vi "Real_Time_State_Machine.vi"() -> ()   [LabVIEW 2019]
uses:
  <vilib>/Platform/TimedLoop/XDataNode/wakeup.ctl
  <vilib>/Platform/TimedLoop/XDataNode/XDNodeRunTimeDep.lvlib
  <vilib>/Platform/TimedLoop/XDataNode/nitl_modes.ctl
  <vilib>/Platform/TimedLoop/XDataNode/timing_clust.ctl
  <vilib>/platform/TimedLoop/XDataNode/XDataNode.xnode
  <vilib>/myRIO/Common/Instrument Driver Framework/myRIO v1.0/Accelerometer/typedefs/Accelerometer Channels Enum.ctl
  <vilib>/myRIO/Common/Instrument Driver Framework/myRIO v1.0/Accelerometer/typedefs/Accelerometer Channels List.ctl
  <vilib>/myRIO/Common/Instrument Driver Framework/Utilities/typedefs/Generic FPGA Reference.ctl
  <vilib>/myRIO/Common/Instrument Driver Framework/Utilities/typedefs/myRIO v1.0 Reference.ctl
  <vilib>/myRIO/Common/Instrument Driver Framework/Utilities/typedefs/Hardware Version Enum.ctl
  <vilib>/myRIO/Common/Instrument Driver Framework/Utilities/typedefs/myRIO Generic Hardware Reference.ctl
  <vilib>/myRIO/Instrument Drivers/Onboard Devices/Accelerometer/typedefs/Accelerometer Reference.ctl
  <vilib>/myRIO/Instrument Drivers/Onboard Devices/Accelerometer/Accelerometer.lvlib
  <vilib>/myRIO/Instrument Drivers/Onboard Devices/Accelerometer/vis/Read.vi
  <vilib>/userDefined/High Color/nirio_resource_hc.ctl
  <vilib>/myRIO/Instrument Drivers/Onboard Devices/Accelerometer/vis/myRIO Accelerometer Open.xnode
  <vilib>/myRIO/Common/Instrument Driver Framework/Utilities/vis/Is FPGA Ref Available.vi
  <vilib>/myRIO/Express VI/Onboard Devices/Accelerometer/Accelerometer Express VI.xnode
  <vilib>/myRIO/Common/Instrument Driver Framework/myRIO v1.0/DIO/typedefs/DIO Channels Enum.ctl
  <vilib>/myRIO/Common/Instrument Driver Framework/myRIO v1.0/DIO/typedefs/DIO Channels List.ctl
  <vilib>/myRIO/Instrument Drivers/Onboard IO/DIO/typedefs/DIO Reference.ctl
  <vilib>/myRIO/Instrument Drivers/Onboard IO/DIO/DIO.lvlib
  <vilib>/myRIO/Instrument Drivers/Onboard IO/DIO/vis/myRIO DIO Open.xnode
  <vilib>/myRIO/Instrument Drivers/Onboard IO/DIO/vis/Write.vi
  <vilib>/myRIO/Express VI/Onboard Devices/LED/LED Express VI.xnode
  <vilib>/myRIO/Common/Instrument Driver Framework/myRIO v1.0/Accelerometer/vis/myRIO v1.1 Open Accelerometer.vi
  <vilib>/myRIO/Common/Instrument Driver Framework/myRIO v1.0/DIO/vis/myRIO v1.1 Open DIO.vi
  System_State.ctl
  Triggered_State.ctl
  Armed_States.ctl
  Reset_State.ctl
panel:
  in  "Boolean":bool
  in  "Enum 4":T1
  in  "Enum 2":T2
  in  "Enum 3":T3
  in  "Enum":T4=enum."Idle"
  out "Magnitude":dbl
  in  "stop 2":bool
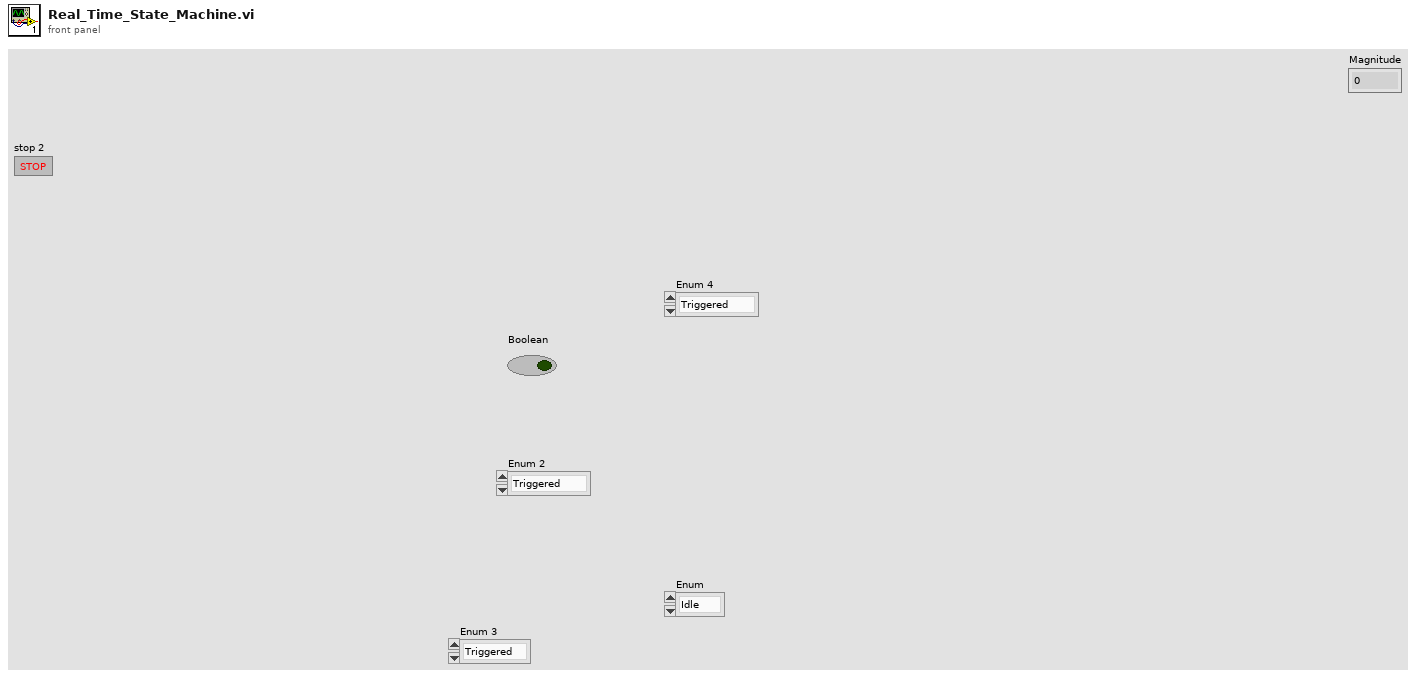
[diagram p1: front panel]
types:
  T1 = typedef "Reset_State.ctl" = enum16{"Triggered", "Armed", "Idle"}
  T2 = typedef "Armed_States.ctl" = enum16{"Triggered", "Armed", "Idle"}
  T3 = typedef "Triggered_State.ctl" = enum16{"Triggered", "Armed", "Idle"}
  T4 = typedef "System_State.ctl" = enum16{"Triggered", "Armed", "Idle"}
  T5 = typedef "XDNodeRunTimeDep.lvlib/timing_clust.ctl" = cluster{"Expected End [f-1]":u64, "Actual End [f-1]":u64, "Finished Late? [f-1]":bool, "Expected End [i-1]":u64, "Actual End [i-1]":u64, "Finished Late? [i-1]":bool, "Expected Start [i]":u64, "Actual Start [i]":u64, "Expected Start [f]":u64, "Actual Start [f]":u64, "Source Name":string, "Structure Name":string, "Period":i64, "Deadline":i64, "Offset":i64, "Start":i64, "Priority":i32, "Timeout":i32, "Mode":T6, "Wakeup Reason":T7, "Error":errorcluster, "Source Type":string, "Secondary Source Type":string, "Global End Time":u64, "Global Start Time":u64, "Frame Duration":u64, "Iteration Duration":u64, "Assigned CPU":i32, "I/O Scan Engine Mode":u32}
  T6 = typedef "XDNodeRunTimeDep.lvlib/nitl_modes.ctl" = enum32{"No Change", "Process missed periods, maintain original phase", "Discard missed periods, maintain original phase", "Process missed periods, ignore original phase", "Discard missed periods, ignore original phase"}
  T7 = typedef "XDNodeRunTimeDep.lvlib/wakeup.ctl" = enum32{"Normal", "Aborted", "Asynchronous wakeup", "Timing source error", "Timed loop error", "Timeout"}
  T8 = typedef "DIO.lvlib/DIO Reference.ctl" = cluster{"myRIO Reference":T9, "DIO Channels List":T13}
  T9 = typedef "myRIO Generic Hardware Reference.ctl" = cluster{"myRIO Model":T10, "myRIO Hardware Reference":T11}
  T10 = typedef "Hardware Version Enum.ctl" = enum16{"Unknown", "myRIO-1900", "myRIO-1950", "roboRIO", "NI ELVIS RIO CM", "ELVIS III"}
  T11 = typedef "myRIO v1.0 Reference.ctl" = cluster{"Generic FPGA Reference":T12, "Allow multiple opens":bool}
  T12 = typedef "Generic FPGA Reference.ctl" = refnum<k20>
  T13 = typedef "DIO Channels List.ctl" = T14[]
  T14 = typedef "DIO Channels Enum.ctl" = enum16{"Not Connected", "C/DIO0", "C/DIO1", "C/DIO2", "C/DIO3", "C/DIO4", "C/DIO5", "C/DIO6", "C/DIO7", "A/DIO0", "A/DIO1", "A/DIO2", "A/DIO3", "A/DIO4", "A/DIO5", "A/DIO6", "A/DIO7", "A/DIO8", "A/DIO9", "A/DIO10", "A/DIO11", "A/DIO12", "A/DIO13", "A/DIO14", "A/DIO15", "A/DIO16", "A/DIO17", "A/DIO18", "A/DIO19", "B/DIO0", "B/DIO1", "B/DIO2", "B/DIO3", "B/DIO4", "B/DIO5", "B/DIO6", "B/DIO7", "B/DIO8", "B/DIO9", "B/DIO10", "B/DIO11", "B/DIO12", "B/DIO13", "B/DIO14", "B/DIO15", "B/DIO16", "B/DIO17", "B/DIO18", "B/DIO19", "LED0", "LED1", "LED2", "LED3", "Button0", "DIO/DIO0", "DIO/DIO1", "DIO/DIO2", "DIO/DIO3", "DIO/DIO4", "DIO/DIO5", "DIO/DIO6", "DIO/DIO7", "DIO/DIO8", "DIO/DIO9", "SPI/CS0", "SPI/CS1", "SPI/CS2", "SPI/CS3", "LED RADIO (Green)", "LED RADIO (Red)", "LED COMM (Green)", "LED COMM (Red)", "LED MODE (Green)", "LED MODE (Red)"}
  T15 = typedef "nirio_resource_hc.ctl" = tag
  T16 = typedef "Accelerometer.lvlib/Accelerometer Reference.ctl" = cluster{"myRIO Reference":T9, "Accelerometer Channels List":T17, "LSB Weight":dbl}
  T17 = typedef "Accelerometer Channels List.ctl" = T18[]
  T18 = typedef "Accelerometer Channels Enum.ctl" = enum16{"Not Connected", "X-Axis", "Y-Axis", "Z-Axis"}
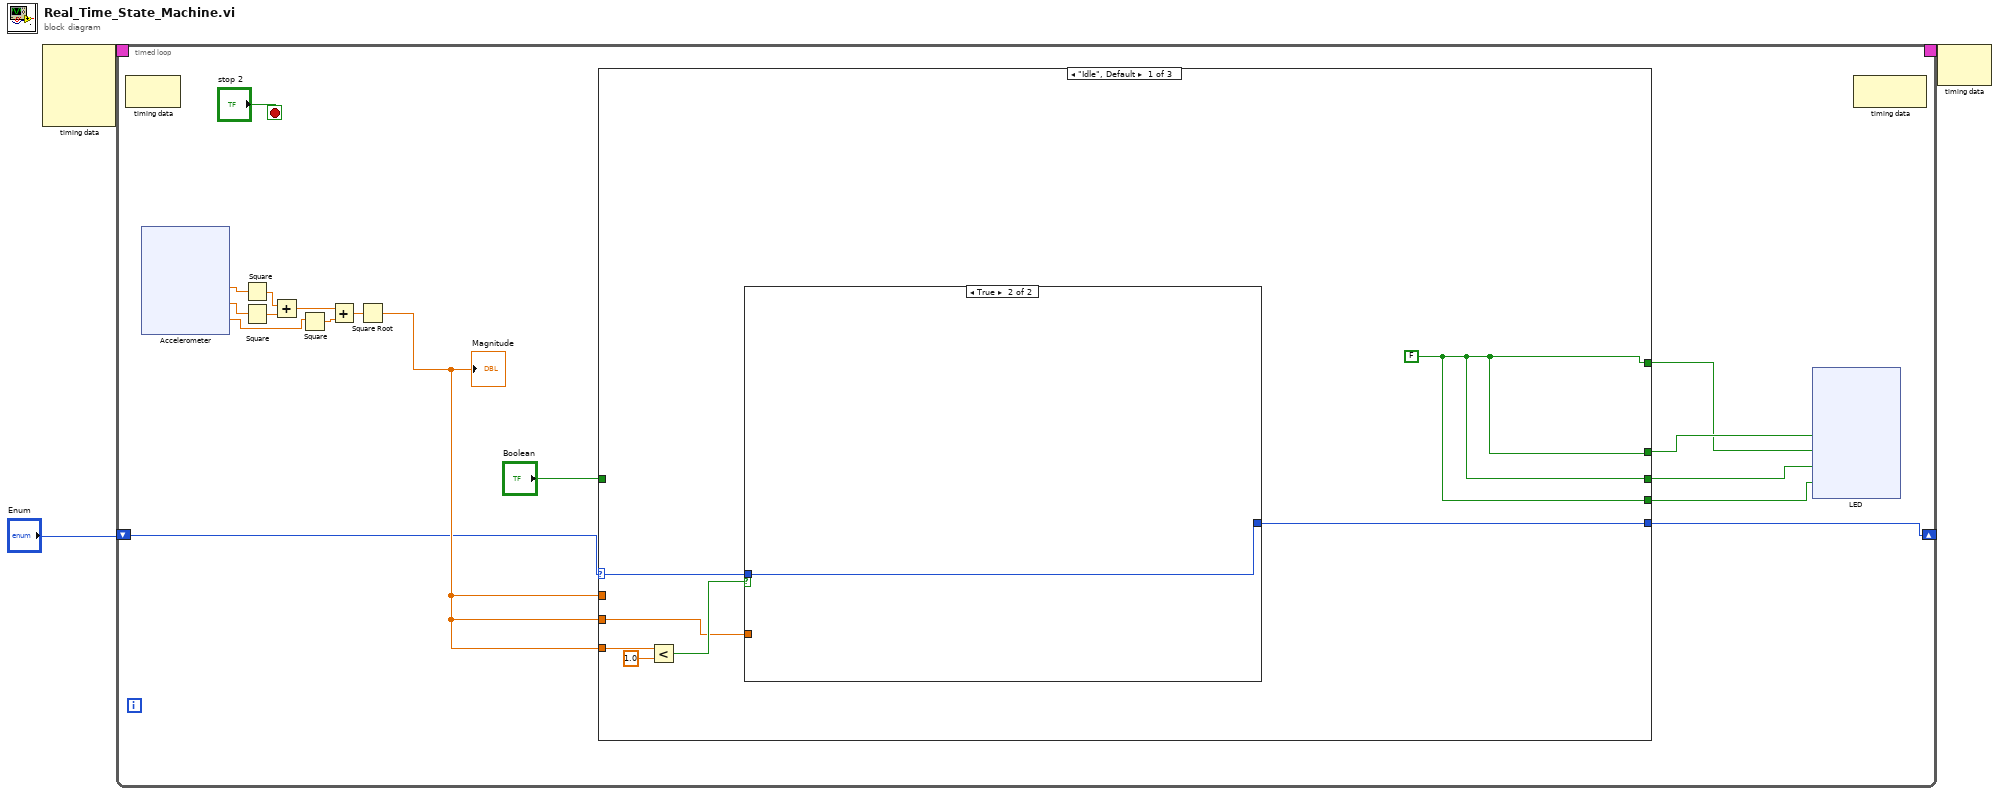
[diagram p0: block diagram]
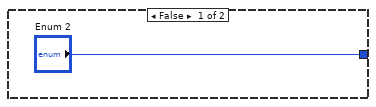
[diagram p2: hidden frame]
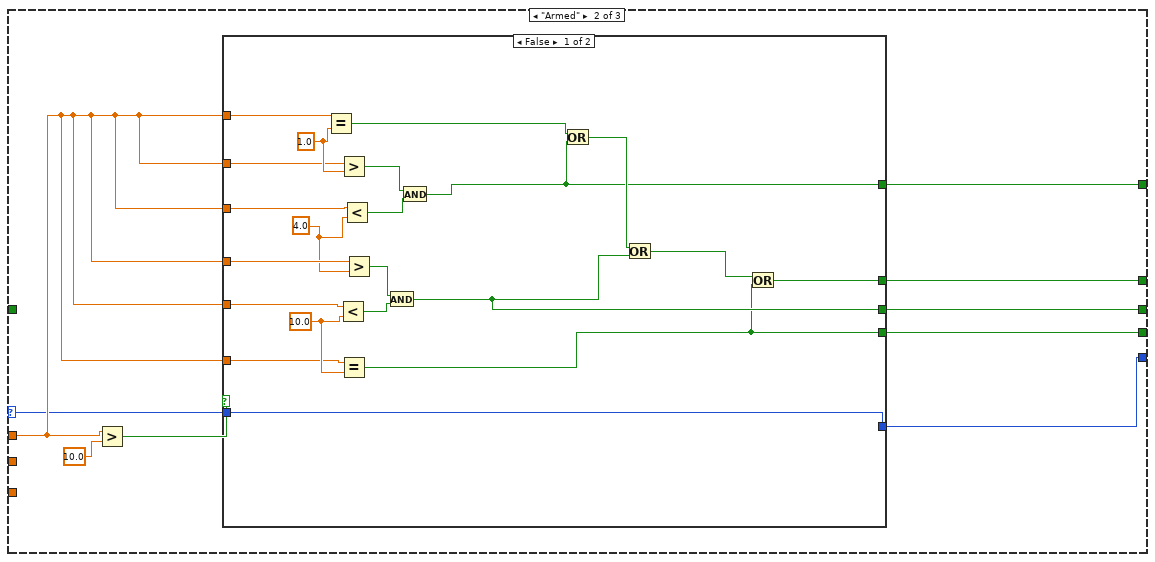
[diagram p3: hidden frame]
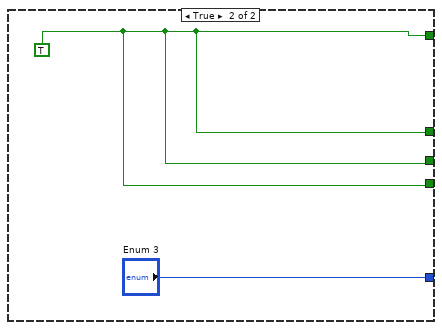
[diagram p4: hidden frame]
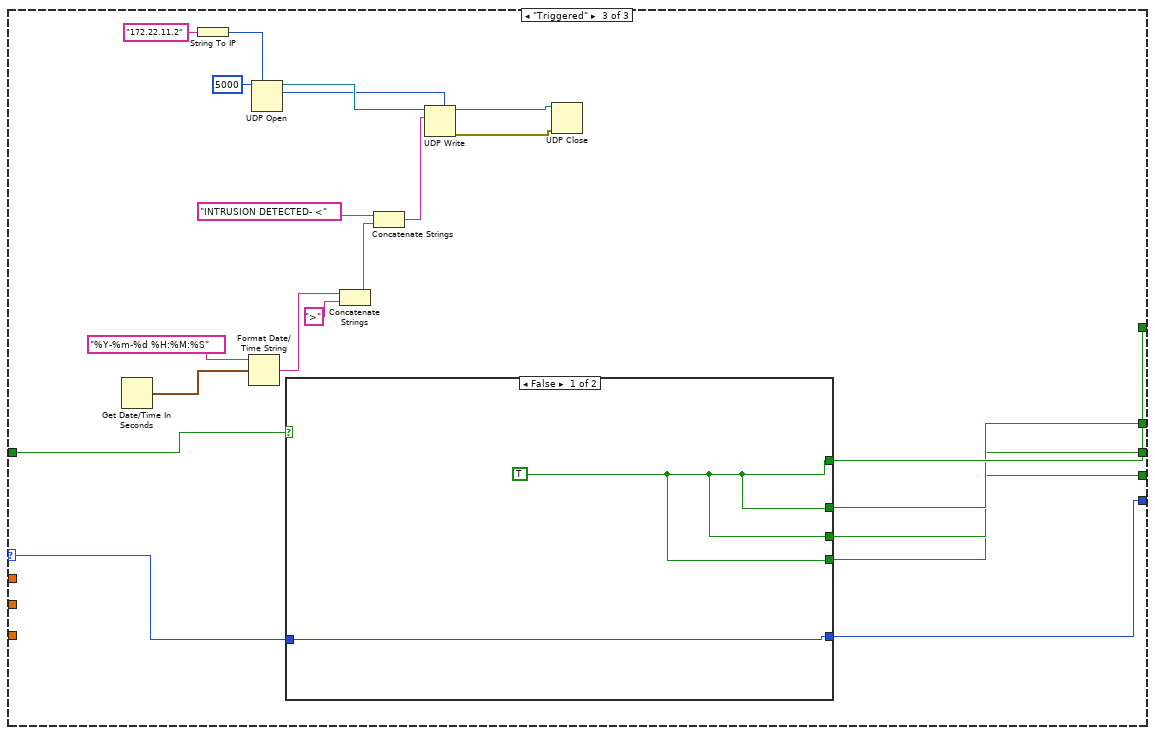
[diagram p5: hidden frame]
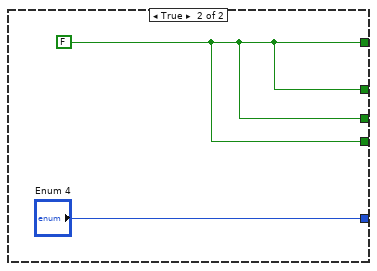
[diagram p6: hidden frame]
diagram:
  n1 = node-c288() -> (w3:T5)  [unwired: 4 in]
  n2 = timed-loop {
    timing: w3 -> [_]
    timing-out: [_] -> w2
    shift-right: [w5] -> _
    shift-left: "Enum" -> [w6]
    stop <- "stop 2" stop-if-true
    n3 = node-c288() -> ()  [unwired: 1 in, 1 out]
    n4 = xnode "Accelerometer"() -> ("X-Axis"=w19:dbl, "Y-Axis"=w18:dbl, "Z-Axis"=w17:dbl)  [unwired: 1 in, 1 out]
    n5 = Square(x=w19) -> (x^2=w16:dbl)
    n6 = Square(x=w18) -> (x^2=w15:dbl)
    n7 = Add(x=w16, y=w15) -> (x+y=w14:dbl)
    n8 = Square(x=w17) -> (x^2=w13:dbl)
    n9 = Add(x=w14, y=w13) -> (x+y=w12:dbl)
    n10 = Square Root(x=w12) -> (sqrt(x)=w11:dbl)
    "Magnitude" <- w11
    n11 = case shown="\"Idle\", Default" w6 {
      selector: w6 -> [w59 w68 w114]
      tunnel: w11 -> [w64 _ _]
      tunnel: w11 -> [w62 _ _]
      tunnel: w11 -> [_ w74 _]
      tunnel: [w61 w73 w118] -> w10
      tunnel: [w61 w72 w119] -> w9
      tunnel: [w61 w71 w117] -> w8
      tunnel: [w61 w70 w116] -> w7
      tunnel: [w60 w69 w115] -> w5
      tunnel: "Boolean" -> [_ _ w120]
      frame "Idle", Default {
        w61 = FALSE
        n12 = Less?(x=w64, y=1.0) -> (x < y?=w63:bool)
        n13 = case shown="True" w63 {
          tunnel: w62 -> [_ _]
          tunnel: ["Enum 2" w67] -> w60
          tunnel: w59 -> [_ w67]
          frame False {
          }
          frame True {
          }
        }
      }
      frame "Armed" {
        n14 = Greater?(x=w74, y=10.0) -> (0:w75:bool)
        n15 = case shown="False" w75 {
          tunnel: w74 -> [w97 _]
          tunnel: w74 -> [w95 _]
          tunnel: w74 -> [w91 _]
          tunnel: w74 -> [w94 _]
          tunnel: w74 -> [w88 _]
          tunnel: w74 -> [w85 _]
          tunnel: [w81 w99] -> w73
          tunnel: [w80 w99] -> w72
          tunnel: [w79 w99] -> w71
          tunnel: [w78 w99] -> w70
          tunnel: [w77 "Enum 3"] -> w69
          tunnel: w68 -> [w77 _]
          frame False {
            w86 = 10.0 ("y")
            w90 = 4.0 ("y")
            w96 = 1.0 ("y")
            n16 = Equal?(x=w97, y=w96) -> (x = y?=w84:bool)
            n17 = Less?(x=w88, y=w86) -> (x < y?=w87:bool)
            n18 = Greater?(x=w95, y=w96) -> (0:w93:bool)
            n19 = Equal?(x=w85, y=w86) -> (x = y?=w78:bool)
            n20 = Less?(x=w91, y=w90) -> (x < y?=w89:bool)
            n21 = Greater?(x=w94, y=w90) -> (0:w92:bool)
            n22 = And(x=w92, y=w87) -> (x .and. y?=w79:bool)
            n23 = And(x=w93, y=w89) -> (x .and. y?=w80:bool)
            n24 = Or(x=w84, y=w80) -> (x .or. y?=w83:bool)
            n25 = Or(x=w83, y=w79) -> (x .or. y?=w82:bool)
            n26 = Or(x=w82, y=w78) -> (x .or. y?=w81:bool)
          }
          frame True {
            w99 = TRUE
          }
        }
      }
      frame "Triggered" {
        n27 = Get Date/Time In Seconds() -> (seconds since 1Jan1904=w110:timestamp)
        n28 = String To IP(1:"172.22.11.2" ("name")) -> (0:w111:u32)
        n29 = Format Date/Time String(time format string (%c)="%Y-%m-%d %H:%M:%S", seconds (now)=w110) -> (date/time string=w104:string)  [unwired: 1 in]
        n30 = UDP Open(7:w111, 11:u16 5000 ("port")) -> (port=w108:refnum<k16>, 2:w107:u16)  [unwired: 3 in, 1 out]
        n31 = case shown="False" w120 {
          tunnel: [w121 w124] -> w119
          tunnel: [w121 w124] -> w118
          tunnel: [w121 w124] -> w117
          tunnel: [w121 w124] -> w116
          tunnel: [w122 "Enum 4"] -> w115
          tunnel: w114 -> [w122 _]
          frame False {
            w121 = TRUE
          }
          frame True {
            w124 = FALSE
          }
        }
        n32 = Concatenate Strings(w104, ">" ("string")) -> (w102:string)
        n33 = Concatenate Strings("INTRUSION DETECTED- <" ("string"), w102) -> (w101:string)
        n34 = UDP Write(port or service name=w107, connection ID=w108, data in=w101) -> (error out=w106:errorcluster, 3:w100:refnum<k16>)  [unwired: 3 in]
        n35 = UDP Close(connection ID=w100, 8:w106) -> ()  [unwired: 2 out]
      }
    }
    n36 = xnode "LED"("LED0"=w10, "LED1"=w9, "LED2"=w8, "LED3"=w7) -> ()  [unwired: 1 in, 1 out]
    n37 = node-c288() -> ()  [unwired: 1 in, 1 out]
  }
  n38 = node-c288(w2) -> ()  [unwired: 1 out]
